vi "swerve_periodic.vi"(8 "Field Oriented?":bool, 9 "Rotate":dbl(slide) scale=-1.0..1.0, 10 "Forwards":dbl(slide) scale=-1.0..1.0, 11 "Strafe":dbl(slide) scale=-1.0..1.0) -> ()   [LabVIEW 2020]
uses:
  <vilib>/Rock Robotics/WPI/ThirdParty/Phoenix-LabVIEW/Motor Controller/Controls/CTRE_Phoenix_MotorControl_ControlMode.ctl
  swerve_globals.vi
  <vilib>/Rock Robotics/WPI/ThirdParty/Phoenix-LabVIEW/Motor Controller/Get/CTRE_Phoenix_MotorController_GetSelectedSensorData.vi
  TitanLib/Lib/TitanLib.lvlib
panel:
  out "Pose Estimation (in)":cluster{"Pose[0]":dbl, "Pose[1]":dbl}[](graph)
  in  "wheel offset (in)":dbl format="%_6g"
  in  "Reset Odometry?":bool
  in  "Drive Speed Multiplier":dbl=1.0
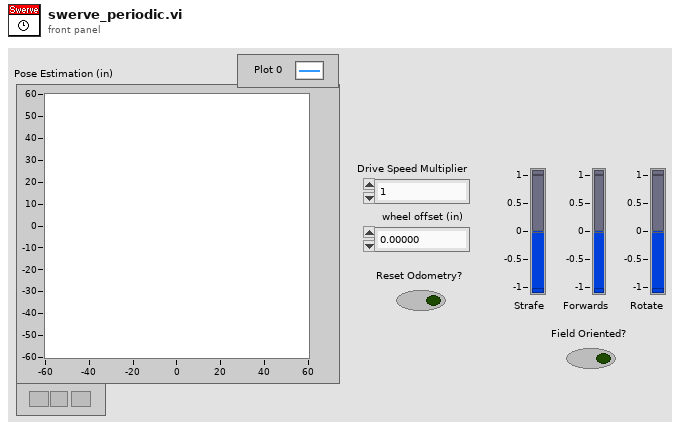
[diagram p1: front panel]
types:
  T1 = typedef "CTRE_Phoenix_MotorControl_ControlMode.ctl" = u16
  T2 = typedef "WPI_MotorControlDeviceRef.ctl" = cluster{"DeviceStatus":errorcluster, "Type":T3, "PWM":cluster{"PWM Channel":T4, "DeadBand":T5}, "CAN":cluster{"Device Number":u8, "SetOutput VI Ref":variant, "GetOutput VI Ref":variant, "Enable VI Ref":variant, "Disable VI Ref":variant, "Data":variant}, "Invert":bool, "DIO PWM":cluster{"PWM \"Enable\" Channel":T4, "DIOChannel":T6, "PWM Rate":dbl}}
  T3 = typedef "WPI_MotorControlType.ctl" = enum16{"PWM", "CAN", "DIO PWM"}
  T4 = typedef "FPGA_DIOPWMChannel.ctl" = enum8{"PWM 0", "PWM 1", "PWM 2", "PWM 3", "PWM 4", "PWM 5", "PWM 6", "PWM 7", "PWM 8", "PWM 9", "PWM MXP 0", "PWM MXP 1", "PWM MXP 2", "PWM MXP 3", "PWM MXP 4", "PWM MXP 5", "PWM MXP 6", "PWM MXP 7", "PWM MXP 8", "PWM MXP 9", "Invalid"}
  T5 = typedef "WPI_PWMDeadband.ctl" = cluster{"Name":string, "maxPositivePwm":i32, "minPositivePwm":i32, "centerPwm":i32, "maxNegativePwm":i32, "minNegativePwm":i32, "angularRange":u16}
  T6 = typedef "FPGA_DIOChannel.ctl" = enum8{"DIO 0", "DIO 1", "DIO 2", "DIO 3", "DIO 4", "DIO 5", "DIO 6", "DIO 7", "DIO 8", "DIO 9", "DIO MXP 0", "DIO MXP 1", "DIO MXP 2", "DIO MXP 3", "DIO MXP 4", "DIO MXP 5", "DIO MXP 6", "DIO MXP 7", "DIO MXP 8", "DIO MXP 9", "DIO MXP 10", "DIO MXP 11", "DIO MXP 12", "DIO MXP 13", "DIO MXP 14", "DIO MXP 15", "SPI Port CS1", "SPI Port CS2", "SPI Port CS3", "SPI Port MISO", "SPI Port MOSI", "Invalid"}
  T7 = typedef "NI_Matrix.lvlib/RealMatrix.ctl" = dbl[][]
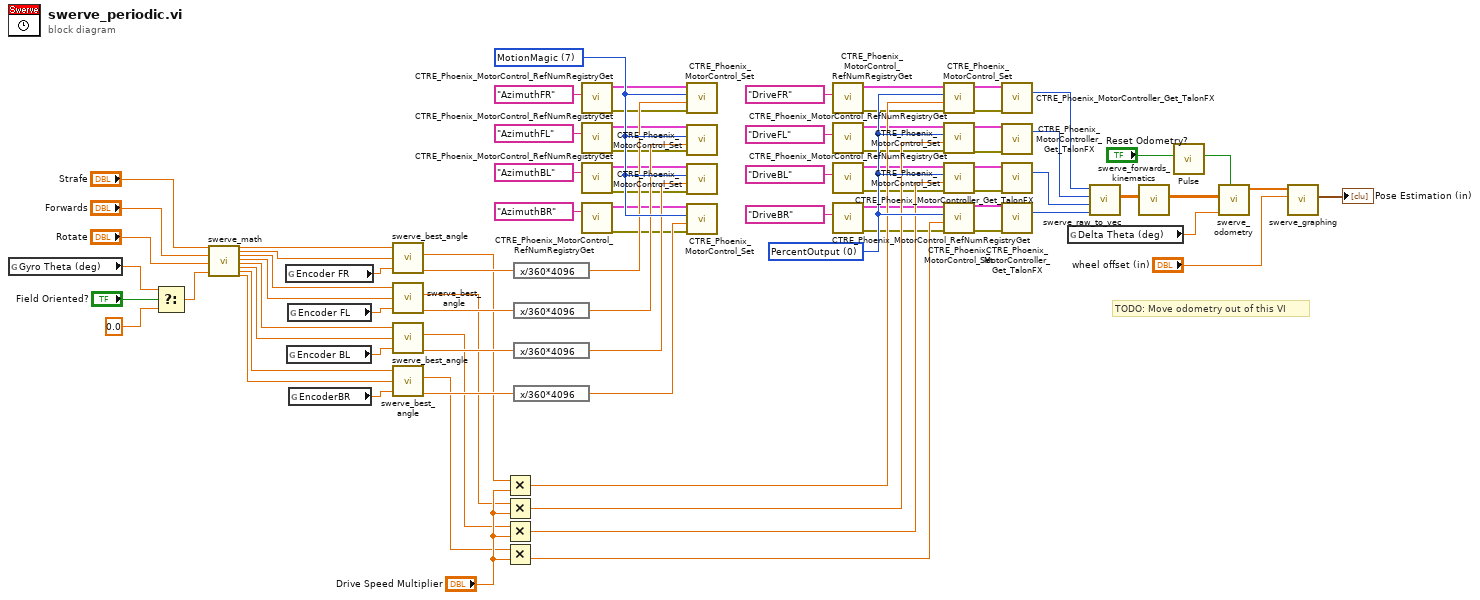
[diagram p0: block diagram]
diagram:
  w68 = T1 0 items=["PercentOutput"=0, "Position"=1, "Velocity"=2, "Current"=3, "Follower"=5, "MotionProfile"=6, "MotionMagic"=7, "MotionProfileArc"=10, "Disabled"=15] ("Control Mode")
  w82 = T1 7 items=["PercentOutput"=0, "Position"=1, "Velocity"=2, "Current"=3, "Follower"=5, "MotionProfile"=6, "MotionMagic"=7, "MotionProfileArc"=10, "Disabled"=15] ("Control Mode")
  # "TODO: Move odometry out of this VI"
  n1 = global read "swerve_globals.vi" "Gyro Theta (deg)"() -> (w8:dbl)
  n2 = Select(t=w8, s="Field Oriented?", f=0.0) -> (s? t:f=w6:dbl)
  n3 = call "swerve_math.vi"("Strafe"="Strafe", "Forwards"="Forwards", "Rotate"="Rotate", "Gyro"=w6) -> ("Drive FR"=w20:dbl, "Azimuth FR"=w15:dbl, "Drive FL"=w14:dbl, "Azimuth FL"=w13:dbl, "Drive BL"=w12:dbl, "Azimuth BL"=w11:dbl, "Drive BR"=w10:dbl, "Azimuth BR"=w9:dbl)  [unwired: 16 in]
  n4 = global read "swerve_globals.vi" "Encoder FR"() -> (w19:dbl)
  n5 = global read "swerve_globals.vi" "Encoder BL"() -> (w17:dbl)
  n6 = global read "swerve_globals.vi" "Encoder FL"() -> (w18:dbl)
  n7 = global read "swerve_globals.vi" "EncoderBR"() -> (w16:dbl)
  n8 = call "swerve_best_angle.vi"("Current Angle"=w19, "Target Angle"=w15, "Power In"=w20) -> ("Setpoint Angle"=w81:dbl, "Power Out"=w72:dbl)  [unwired: 4 in]
  n9 = call "swerve_best_angle.vi"("Current Angle"=w18, "Target Angle"=w13, "Power In"=w14) -> ("Setpoint Angle"=w80:dbl, "Power Out"=w71:dbl)  [unwired: 4 in]
  n10 = call "swerve_best_angle.vi"("Current Angle"=w17, "Target Angle"=w11, "Power In"=w12) -> ("Setpoint Angle"=w79:dbl, "Power Out"=w70:dbl)  [unwired: 4 in]
  n11 = call "swerve_best_angle.vi"("Current Angle"=w16, "Target Angle"=w9, "Power In"=w10) -> ("Setpoint Angle"=w78:dbl, "Power Out"=w69:dbl)  [unwired: 4 in]
  n12 = Multiply(x=w72, y="Drive Speed Multiplier") -> (x*y=w53:dbl)
  n13 = Multiply(x=w71, y="Drive Speed Multiplier") -> (x*y=w52:dbl)
  n14 = Multiply(x=w70, y="Drive Speed Multiplier") -> (x*y=w51:dbl)
  n15 = Multiply(x=w69, y="Drive Speed Multiplier") -> (x*y=w50:dbl)
  n16 = expression code="x/360*4096"(w81) -> (w77:dbl)
  n17 = expression code="x/360*4096"(w80) -> (w76:dbl)
  n18 = expression code="x/360*4096"(w79) -> (w75:dbl)
  n19 = expression code="x/360*4096"(w78) -> (w74:dbl)
  n20 = call <vilib>:"CTRE_Phoenix_MotorControl_RefNumRegistryGet.vi"("refnum name"="AzimuthFR") -> ("error out"=w44:errorcluster, "PhoenixMotorControlDevRef"=w45:T2)  [unwired: 9 in]
  n21 = call <vilib>:"CTRE_Phoenix_MotorControl_RefNumRegistryGet.vi"("refnum name"="AzimuthFL") -> ("error out"=w42:errorcluster, "PhoenixMotorControlDevRef"=w43:T2)  [unwired: 9 in]
  n22 = call <vilib>:"CTRE_Phoenix_MotorControl_RefNumRegistryGet.vi"("refnum name"="AzimuthBL") -> ("error out"=w40:errorcluster, "PhoenixMotorControlDevRef"=w41:T2)  [unwired: 9 in]
  n23 = call <vilib>:"CTRE_Phoenix_MotorControl_RefNumRegistryGet.vi"("refnum name"="AzimuthBR") -> ("error out"=w38:errorcluster, "PhoenixMotorControlDevRef"=w39:T2)  [unwired: 9 in]
  n24 = call <vilib>:"CTRE_Phoenix_MotorControl_Set.vi"("error in (no error)"=w44, "Output"=w77, "Control Mode"=w82, "PhoenixMotorControlDevRef"=w45) -> ()  [unwired: 6 in, 2 out]
  n25 = call <vilib>:"CTRE_Phoenix_MotorControl_Set.vi"("error in (no error)"=w42, "Output"=w76, "Control Mode"=w82, "PhoenixMotorControlDevRef"=w43) -> ()  [unwired: 6 in, 2 out]
  n26 = call <vilib>:"CTRE_Phoenix_MotorControl_Set.vi"("error in (no error)"=w40, "Output"=w75, "Control Mode"=w82, "PhoenixMotorControlDevRef"=w41) -> ()  [unwired: 6 in, 2 out]
  n27 = call <vilib>:"CTRE_Phoenix_MotorControl_Set.vi"("error in (no error)"=w38, "Output"=w74, "Control Mode"=w82, "PhoenixMotorControlDevRef"=w39) -> ()  [unwired: 6 in, 2 out]
  n28 = call <vilib>:"CTRE_Phoenix_MotorControl_RefNumRegistryGet.vi"("refnum name"="DriveFR") -> ("error out"=w26:errorcluster, "PhoenixMotorControlDevRef"=w27:T2)  [unwired: 9 in]
  n29 = call <vilib>:"CTRE_Phoenix_MotorControl_RefNumRegistryGet.vi"("refnum name"="DriveFL") -> ("error out"=w28:errorcluster, "PhoenixMotorControlDevRef"=w29:T2)  [unwired: 9 in]
  n30 = call <vilib>:"CTRE_Phoenix_MotorControl_RefNumRegistryGet.vi"("refnum name"="DriveBL") -> ("error out"=w30:errorcluster, "PhoenixMotorControlDevRef"=w31:T2)  [unwired: 9 in]
  n31 = call <vilib>:"CTRE_Phoenix_MotorControl_RefNumRegistryGet.vi"("refnum name"="DriveBR") -> ("error out"=w32:errorcluster, "PhoenixMotorControlDevRef"=w33:T2)  [unwired: 9 in]
  n32 = call <vilib>:"CTRE_Phoenix_MotorControl_Set.vi"("error in (no error)"=w26, "Output"=w53, "Control Mode"=w68, "PhoenixMotorControlDevRef"=w27) -> ("error out"=w66:errorcluster, "PhoenixMotorControlDevRef"=w67:T2)  [unwired: 6 in]
  n33 = call <vilib>:"CTRE_Phoenix_MotorControl_Set.vi"("error in (no error)"=w28, "Output"=w52, "Control Mode"=w68, "PhoenixMotorControlDevRef"=w29) -> ("error out"=w64:errorcluster, "PhoenixMotorControlDevRef"=w65:T2)  [unwired: 6 in]
  n34 = call <vilib>:"CTRE_Phoenix_MotorControl_Set.vi"("error in (no error)"=w30, "Output"=w51, "Control Mode"=w68, "PhoenixMotorControlDevRef"=w31) -> ("error out"=w62:errorcluster, "PhoenixMotorControlDevRef"=w63:T2)  [unwired: 6 in]
  n35 = call <vilib>:"CTRE_Phoenix_MotorControl_Set.vi"("error in (no error)"=w32, "Output"=w50, "Control Mode"=w68, "PhoenixMotorControlDevRef"=w33) -> ("error out"=w60:errorcluster, "PhoenixMotorControlDevRef"=w61:T2)  [unwired: 6 in]
  n36 = call-poly <vilib>:"CTRE_Phoenix_MotorController_Get_TalonFX.vi"("PhoenixMotorControlDevRef"=w67, "error in"=w66) -> ("Position (Raw Sensor Units)"=w58:i32)  [unwired: 10 in, 3 out]
  n37 = call-poly <vilib>:"CTRE_Phoenix_MotorController_Get_TalonFX.vi"("PhoenixMotorControlDevRef"=w65, "error in"=w64) -> ("Position (Raw Sensor Units)"=w57:i32)  [unwired: 10 in, 3 out]
  n38 = call-poly <vilib>:"CTRE_Phoenix_MotorController_Get_TalonFX.vi"("PhoenixMotorControlDevRef"=w63, "error in"=w62) -> ("Position (Raw Sensor Units)"=w56:i32)  [unwired: 10 in, 3 out]
  n39 = call-poly <vilib>:"CTRE_Phoenix_MotorController_Get_TalonFX.vi"("PhoenixMotorControlDevRef"=w61, "error in"=w60) -> ("Position (Raw Sensor Units)"=w23:i32)  [unwired: 10 in, 3 out]
  n40 = global read "swerve_globals.vi" "Delta Theta (deg)"() -> (w24:dbl)
  n41 = call "swerve_raw_to_vec.vi"("Raw Position BR"=w23, "Raw Position BL"=w56, "Raw Position FL"=w57, "Raw Position FR"=w58) -> ("Output Vector"=w22:T7)  [unwired: 7 in]
  n42 = call "swerve_forwards_kinematics.vi"("Input Vector"=w22) -> ("Output Vector"=w55:T7)  [unwired: 10 in]
  n43 = call "Pulse.vi"("Input"="Reset Odometry?") -> ("Output"=w5:bool)  [unwired: 10 in]
  n44 = call "swerve_odometry.vi"("Reset?"=w5, "Delta Theta (deg)"=w24, "input vector"=w55) -> ("Pose"=w54:dbl[])  [unwired: 8 in]
  n45 = call "swerve_graphing.vi"("wheel offset"="wheel offset (in)", "Pose"=w54) -> ("Output"=→"Pose Estimation (in)":cluster{"x out":dbl, "y out":dbl}[])  [unwired: 9 in]
